vi "Get Actual Torque.vi"(8 "error in":errorcluster, 10 "MCU Selector":T1, 11 "HSU MCU V2 Monitor CFG in":refnum<class "HSU MCU V2 CFG.lvclass">) -> (0 "error out":errorcluster, 2 "Torque":dbl format="%#_g Nm", 3 "HSU MCU V2 Monitor CFG out":refnum<class "HSU MCU V2 CFG.lvclass">)   [LabVIEW 2024, in "HSU MCU V2 CFG.lvclass"]
uses:
  HSU MCU V2 CFG.lvclass
  MCU Selector.ctl
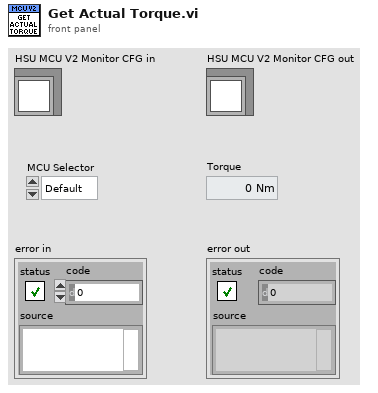
[diagram p1: front panel]
types:
  T1 = typedef "MCU Selector.ctl" = enum16{"Default", "MCU1", "MCU2", "MCU3", "MCU4", "MCU5", "MCU6", "MCU7", "MCU8", "ALL"}
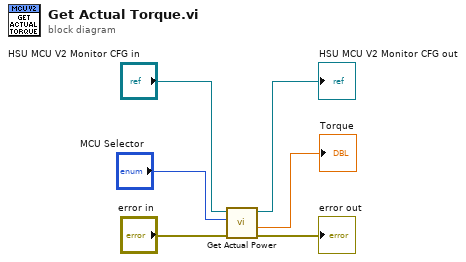
[diagram p0: block diagram]
diagram:
  n1 = call "Get Actual Power.vi"("error in"="error in", 10:"MCU Selector", "HSU MCU V2 CFG in"="HSU MCU V2 Monitor CFG in") -> ("error out"=→"error out":errorcluster, "Torque"=→"Torque":dbl, "HSU MCU V2 CFG out"=→"HSU MCU V2 Monitor CFG out":refnum<class "HSU MCU V2 CFG.lvclass">)  [unwired: 5 in, 1 out]
